vi "Run.vi"(7 "Team Index":i32, 8 "Column":i32, 9 "Row":i32, 10 "View":i32[](array[numeric]) caption="View (Team Index, -1: empty)", 11 "Runner in":refnum<class "AntFarm_MB.lvclass">) -> (0 "Replicated":refnum<class "Square.lvclass">, 1 "Direction":T1, 2 "Action":T2, 3 "Square Out":refnum<class "Square.lvclass">)   [LabVIEW 2017, in "AntFarm_MB.lvclass"]
uses:
  AntFarm_MB.lvclass
  C:/GIT/Endigit/SquareBattle/Square/Square.lvclass
  Square/Square.lvclass
  Type Defs/Action Enum.ctl
  Type Defs/Direction Enum.ctl
  AntFarm_MB.lvclass/AntFarm_MB.ctl
  TypeDefs/Cluster_Square Data.ctl
  TypeDefs/ENUM_Position ID.ctl
  Type Defs/SB Type Defs.lvlib
panel:
  out "New View Out":i32[](array[numeric])
  # "NW\nN\nNE\nE\nSE\nS\nSW\nW"
  # "NOTICE - YOU MUST NOT REMOVE THIS NOTICE. PER THE FOLLOWING LICENSE, YOU MAY REPRODUCE THIS SOFTWARE PROVIDED YOU FOLLOW THE TERMS\nOF THE LICENSE.\n\n---BEGIN BSD LICENSE (http://opensource.org/licenses/BSD-2-Clause)---\nCopyright (c) 2015, Endigit, Inc. <robert@endigit.com>\nAll rights reserved.\n\nRedistribution and use in source and binary forms, with or without modification, are permitted provided that the following conditions are met:\n\n1. Redistributions of source code must retain the above copyright notice, this list of conditions and the following disclaimer.\n\n2. Redistributions in binary form must reproduce the above copyright notice, this list of conditions and the following disclaimer in the documentation and/or other \nmaterials provided with the distribution.\n\nTHIS SOFTWARE IS PROVIDED BY THE COPYRIGHT HOLDERS AND CONTRIBUTORS \"AS IS\" AND ANY EXPRESS OR IMPLIED WARRANTIES, INCLUDING, BUT NOT \nLIMITED TO, THE IMPLIED WARRANTIES OF MERCHANTABILITY AND FITNESS FOR A PARTICULAR PURPOSE ARE DISCLAIMED. IN NO EVENT SHALL THE COPYRIGHT \nHOLDER OR CONTRIBUTORS BE LIABLE FOR ANY DIRECT, INDIRECT, INCIDENTAL, SPECIAL, EXEMPLARY, OR CONSEQUENTIAL DAMAGES (INCLUDING, BUT NOT \nLIMITED TO, PROCUREMENT OF SUBSTITUTE GOODS OR SERVICES; LOSS OF USE, DATA, OR PROFITS; OR BUSINESS INTERRUPTION) HOWEVER CAUSED AND ON \nANY THEORY OF LIABILITY, WHETHER IN CONTRACT, STRICT LIABILITY, OR TORT (INCLUDING NEGLIGENCE OR OTHERWISE) ARISING IN ANY WAY OUT OF THE USE \nOF THIS SOFTWARE, EVEN IF ADVISED OF THE POSSIBILITY OF SUCH DAMAGE.\n---END BSD LICENSE---"
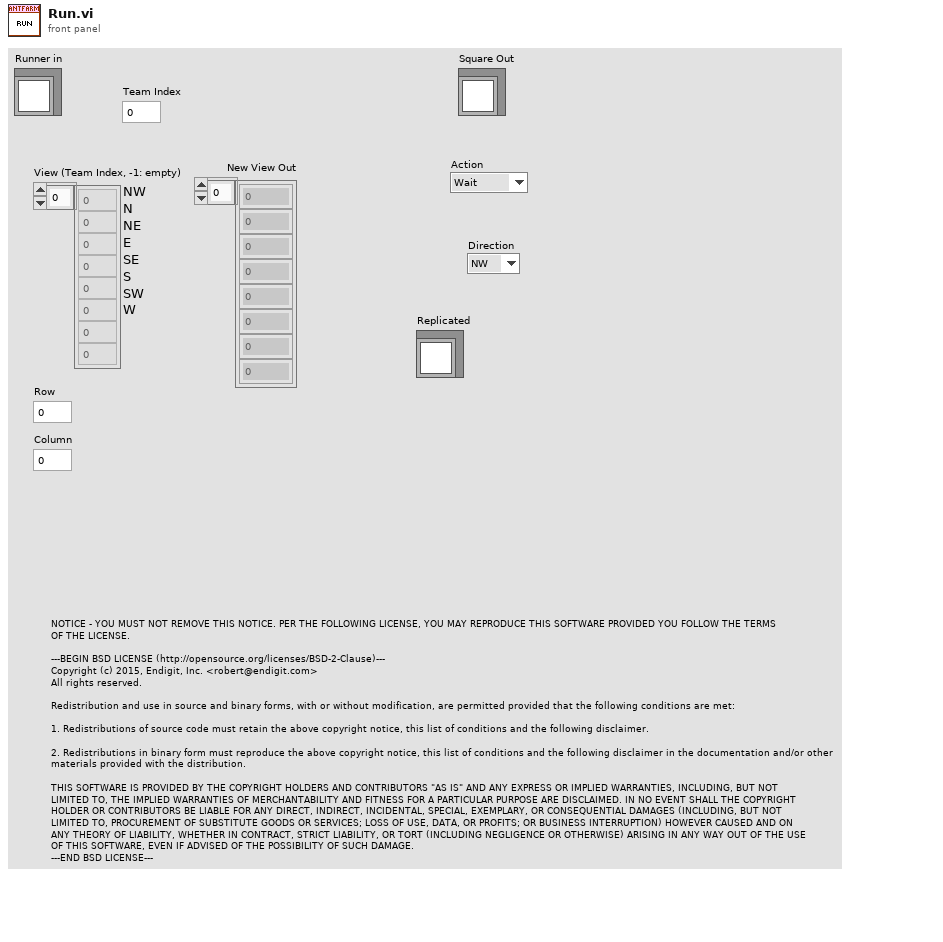
[diagram p1: front panel]
types:
  T1 = typedef "SB Type Defs.lvlib/Direction Enum.ctl" = enum16{"NW", "N", "NE", "E", "SE", "S", "SW", "W"}
  T2 = typedef "SB Type Defs.lvlib/Action Enum.ctl" = enum16{"Wait", "Move", "Attack", "Replicate"}
  T3 = typedef "Cluster_Square Data.ctl" = cluster{"Row":i32, "Column":i32, "Position ID":T4, "Primary Direction":T1, "Action":T2, "Direction":T1, "View":i32[], "New View Out":i32[], "Order ID":i32}
  T4 = typedef "ENUM_Position ID.ctl" = enum16{"0-0 Queen SW", "0-1 Path E", "0-2 Queen NW", "0-3 Path W", "1-0 Path S", "1-1 Larva SW", "1-2 Path N", "1-3 Larva NW", "2-0 Queen SE", "2-1 Path W", "2-2 Queen NE", "2-3 Path E", "3-0 Path N", "3-1 Larva SE", "3-2 Path S", "3-3 Larva NE"}
  T5 = typedef "Cluster_Ant Farm Global Data.ctl" = cluster{"Move Map":i32[][], "Danger Map":i32[][], "Attack Rows":i32[], "Attack Columns":i32[], "Square count":i32, "Last Round":i32, "Danger Threshold":i32}
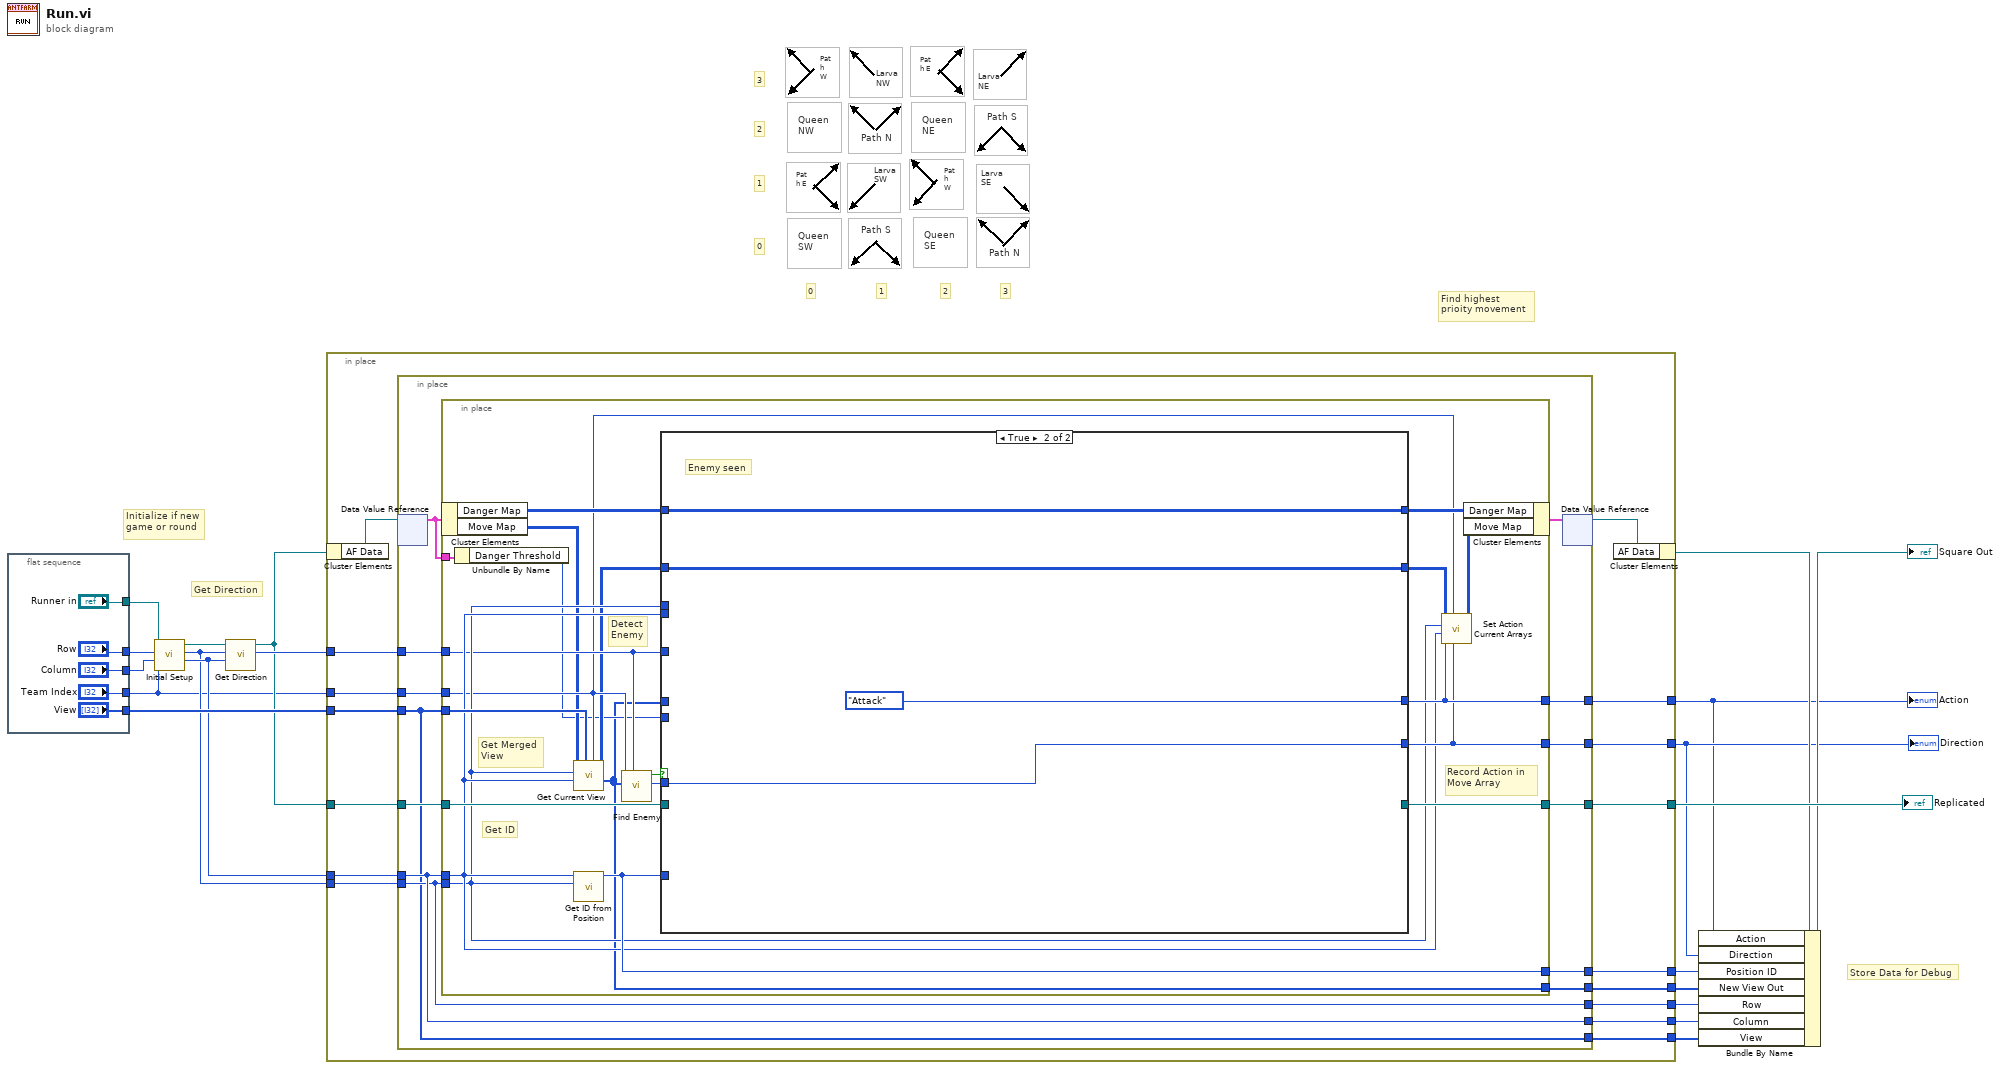
[diagram p0: block diagram]
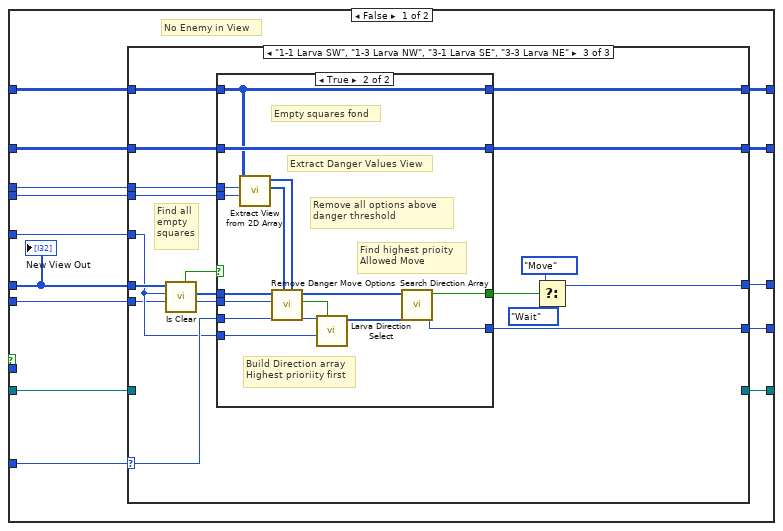
[diagram p2: hidden frame]
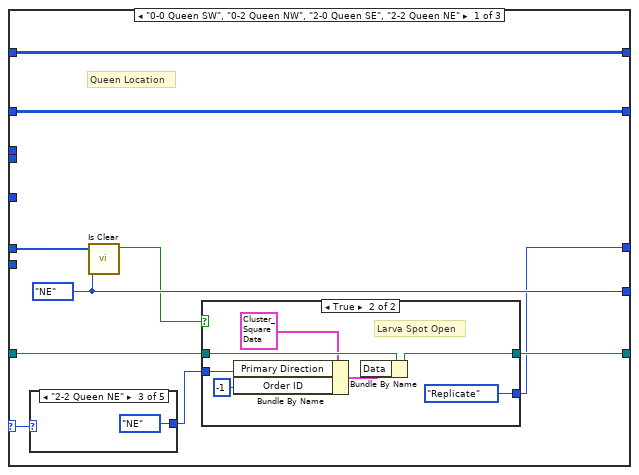
[diagram p3: hidden frame]
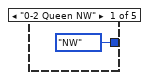
[diagram p4: hidden frame]
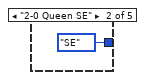
[diagram p5: hidden frame]
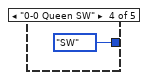
[diagram p6: hidden frame]
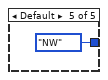
[diagram p7: hidden frame]
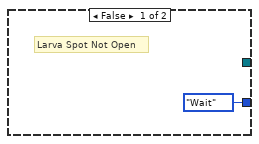
[diagram p8: hidden frame]
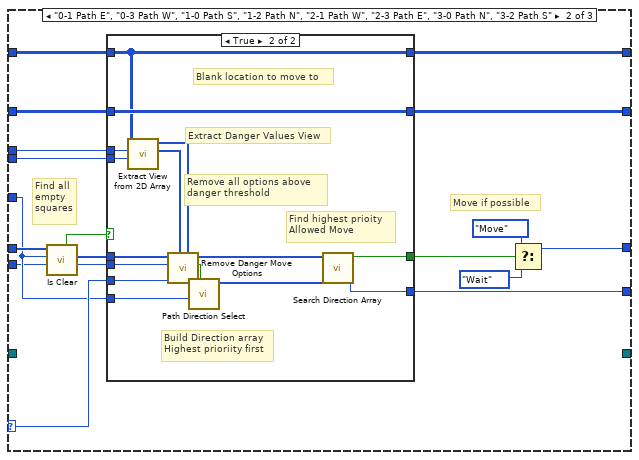
[diagram p9: hidden frame]
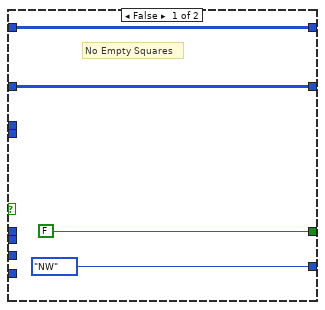
[diagram p10: hidden frame]
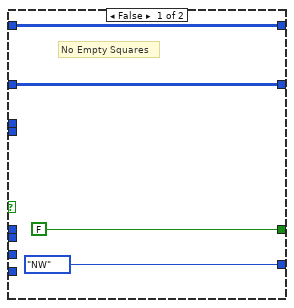
[diagram p11: hidden frame]
diagram:
  # "Store Data for Debug"
  # "Get Direction"
  # "Initialize if new\ngame or round"
  # "Path N"
  # "Path E"
  # "Path S"
  # "Path W"
  # "Path W"
  # "Path S"
  # "Path E"
  # "Path N"
  # "Larva\nNE"
  # "Larva\nSW"
  # "Larva\nNW"
  # "Queen\nNW"
  # "Queen\nNE"
  # "Queen\nSE"
  # "Larva\nSE"
  # "3"
  # "2"
  # "1"
  # "0"
  # "3"
  # "2"
  # "1"
  # "0"
  # "Find highest\nprioity movement"
  # "Queen\nSW"
  n1 = flat-sequence {
    tunnel: ["Team Index"] -> w3
    tunnel: ["View"] -> w19
    tunnel: ["Runner in"] -> w18
    tunnel: ["Row"] -> w5
    tunnel: ["Column"] -> w4
    frame #0 {
    }
  }
  n2 = call "Initial Setup.vi"("Team Index"=w3, "Column"=w4, "Row"=w5, "Runner"=w18) -> ("Column Out"=w7:i32, "Row Out"=w6:i32, "Runner Out"=w9:refnum<class "AntFarm_MB.lvclass">)  [unwired: 5 in]
  n3 = call "Get Direction.vi"("Column"=w7, "Row"=w6, "AntFarm_MB"=w9) -> ("Direction Out"=w10:T1, "AntFarm_MB Out"=w8:refnum<class "AntFarm_MB.lvclass">)  [unwired: 7 in]
  n4 = in-place {
    in-place-border: [w41] -> w20
    in-place-border: w7 -> [w40]
    in-place-border: w6 -> [w39]
    in-place-border: w3 -> [w38]
    in-place-border: w19 -> [w37]
    in-place-border: [w36] -> w11
    in-place-border: [w35] -> w12
    in-place-border: w8 -> [w34]
    in-place-border: [w33] -> w15
    in-place-border: [w32] -> w1
    in-place-border: [w31] -> w2
    in-place-border: [w30] -> w14
    in-place-border: [w29] -> w13
    in-place-border: w10 -> [w26]
    n5 = in-place-cluster #1(w8) -> ("AF Data"=w28:refnum<data-value>)
    n6 = in-place {
      in-place-border: [w54] -> w41
      in-place-border: w40 -> [w47]
      in-place-border: w39 -> [w46]
      in-place-border: w38 -> [w53]
      in-place-border: w37 -> [w43]
      in-place-border: [w52] -> w36
      in-place-border: [w51] -> w35
      in-place-border: w34 -> [w48]
      in-place-border: [w50] -> w33
      in-place-border: [w46] -> w32
      in-place-border: [w47] -> w31
      in-place-border: [w49] -> w30
      in-place-border: [w43] -> w29
      in-place-border: w26 -> [w44]
      n7 = in-place-dvr #2(w28) -> (w42:T5)  [unwired: 1 out]
      n8 = in-place {
        in-place-border: [w73] -> w54
        in-place-border: w53 -> [w60]
        in-place-border: [w72] -> w52
        in-place-border: [w71] -> w51
        in-place-border: [w69] -> w50
        in-place-border: [w55] -> w49
        in-place-border: w43 -> [w68]
        in-place-border: w48 -> [w67]
        in-place-border: w47 -> [w66]
        in-place-border: w46 -> [w65]
        in-place-border: w44 -> [w61]
        in-place-border: w42 -> [w57]
        # "Record Action in \nMove Array"
        # "Detect\nEnemy"
        # "Get Merged\nView"
        # "Get ID"
        n9 = in-place-cluster #3(w42) -> ("Danger Map"=w64:i32[][], "Move Map"=w59:i32[][])
        n10 = Unbundle By Name(w57) -> ("Danger Threshold"=w56:i32)
        n11 = call "Get Current View.vi"("Team Index"=w60, "View"=w68, "Column"=w66, "Row"=w65, "Move Array"=w59) -> ("New View Out"=w55:i32[], "Move Array"=w58:i32[][])  [unwired: 4 in, 1 out]
        n12 = call "Get ID from Position.vi"("Row"=w65, "Column"=w66) -> ("Position ID"=w69:T4)  [unwired: 9 in]
        n13 = call "Find Enemy.vi"("Primary Direction"=w61, "View"=w55, "Team Index"=w60) -> ("Direction"=w74:T1, "Found"=w75:bool)  [unwired: 7 in]
        n14 = case shown="True" w75 {
          tunnel: [w88 Action_Enum."Attack" ("Action")] -> w72
          tunnel: w74 -> [_ w188]
          tunnel: [w89 w188] -> w71
          tunnel: w55 -> [w86 _]
          tunnel: [w87 _] -> w73
          tunnel: w58 -> [w85 w186]
          tunnel: w67 -> [w84 _]
          tunnel: [w83 w186] -> w70
          tunnel: w69 -> [w82 _]
          tunnel: w61 -> [w81 _]
          tunnel: w64 -> [w80 w185]
          tunnel: [w79 w185] -> w62
          tunnel: w66 -> [w78 _]
          tunnel: w65 -> [w77 _]
          tunnel: w56 -> [w76 _]
          frame False {
            # "No Enemy in View"
            n15 = case shown="\"1-1 Larva SW\", \"1-3 Larva NW\", \"3-1 Larva SE\", \"3-3 Larva NE\"" w82 {
              selector: w82 -> [w92 w123 w159]
              tunnel: w86 -> [w99 w129 w165]
              tunnel: [w97 w121 w157] -> w89
              tunnel: [w95 w122 w158] -> w88
              tunnel: [w98 _ _] -> w87
              tunnel: w85 -> [w93 w117 w153]
              tunnel: w84 -> [w94 _ _]
              tunnel: [w93 w116 w152] -> w83
              tunnel: w81 -> [_ w120 w156]
              tunnel: w80 -> [w90 w119 w155]
              tunnel: [w90 w118 w154] -> w79
              tunnel: w78 -> [_ w115 w151]
              tunnel: w77 -> [_ w114 w150]
              tunnel: w76 -> [_ w113 w149]
              frame "0-0 Queen SW", "0-2 Queen NW", "2-0 Queen SE", "2-2 Queen NE" {
                w97 = Direction_Enum."NE" ("Primary Direction")
                # "Queen Location"
                n16 = case shown="\"2-2 Queen NE\"" w92 {
                  tunnel: [Direction_Enum."NW" ("Primary Direction") Direction_Enum."SE" ("Primary Direction") Direction_Enum."NE" ("Primary Direction") Direction_Enum."SW" ("Primary Direction") Direction_Enum."NW" ("Primary Direction")] -> w91
                  frame "0-2 Queen NW" {
                  }
                  frame "2-0 Queen SE" {
                  }
                  frame "2-2 Queen NE" {
                  }
                  frame "0-0 Queen SW" {
                  }
                  frame Default {
                  }
                }
                n17 = call "Is Clear.vi"("Primary Direction"=w97, "View"=w99) -> ("Primary Clear Out"=w96:bool)  [unwired: 7 in, 2 out]
                n18 = case shown="True" w96 {
                  tunnel: [_ w112] -> w98
                  tunnel: w91 -> [_ w107]
                  tunnel: [Action_Enum."Wait" ("Action") Action_Enum."Replicate" ("Action")] -> w95
                  tunnel: w94 -> [_ w110]
                  frame False {
                    # "Larva Spot Not Open"
                  }
                  frame True {
                    # "Larva Spot Open"
                    n19 = Bundle By Name(cluster=T3 {"Row"=0, "Column"=0, "Position ID"=enum."0-0 Queen SW", "Primary Direction"=enum."NW", "Action"=enum."Wait", "Direction"=enum."NW", "View"=[], "New View Out"=[], "Order ID"=0} ("Data"), "Primary Direction"=w107, "Order ID"=-1) -> (w108:T3)
                    n20 = Bundle By Name(cluster=w110, "Data"=w108) -> (w112:refnum<class "AntFarm_MB.lvclass">)
                  }
                }
              }
              frame "0-1 Path E", "0-3 Path W", "1-0 Path S", "1-2 Path N", "2-1 Path W", "2-3 Path E", "3-0 Path N", "3-2 Path S" {
                # "Find all\nempty\nsquares"
                # "Move if possible"
                n21 = call "Is Clear.vi"("Primary Direction"=w120, "View"=w129) -> ("Clear Array Out"=w127:T1[], "Found Out"=w128:bool)  [unwired: 7 in, 1 out]
                n22 = case shown="True" w128 {
                  tunnel: w127 -> [_ w138]
                  tunnel: [Direction_Enum."NW" ("Seconday Move Direction Out") w147] -> w121
                  tunnel: [FALSE w146] -> w126
                  tunnel: w123 -> [_ w148]
                  tunnel: w120 -> [_ w145]
                  tunnel: [w131 w143] -> w118
                  tunnel: w119 -> [w131 w143]
                  tunnel: w117 -> [w130 w144]
                  tunnel: [w130 w144] -> w116
                  tunnel: w115 -> [_ w134]
                  tunnel: w114 -> [_ w142]
                  tunnel: w113 -> [_ w139]
                  frame False {
                    # "No Empty Squares"
                  }
                  frame True {
                    # "Blank location to move to"
                    # "Build Direction array\nHighest prioriity first"
                    # "Extract Danger Values View"
                    # "Find highest prioity \nAllowed Move"
                    # "Remove all options above \ndanger threshold"
                    n23 = call "Extract View from 2D Array.vi"("Column"=w134, "Row"=w142, "Board Array"=w143) -> ("View Out"=w141:i32[], "Directions Out"=w140:T1[])  [unwired: 7 in]
                    n24 = call "Remove Danger Move Options.vi"("Danger Directions"=w140, "Danger View"=w141, "Danger Threshold"=w139, "Direction List"=w138) -> ("Danger"=w135:bool, "Safe Directions Out"=w137:T1[])  [unwired: 6 in]
                    n25 = call "Path Direction Select.vi"("Danger"=w135, "Target Direction"=w145, "Position ID"=w148) -> ("Direction Array"=w136:T1[])  [unwired: 8 in]
                    n26 = call "Search Direction Array.vi"("Target Items"=w136, "Search Array"=w137) -> ("Found Direction"=w147:T1, "Found"=w146:bool)  [unwired: 8 in]
                  }
                }
                n27 = Select(t=Action_Enum."Move" ("Action"), s=w126, f=Action_Enum."Wait") -> (s? t:f=w122:T2)
              }
              frame "1-1 Larva SW", "1-3 Larva NW", "3-1 Larva SE", "3-3 Larva NE" {
                # "Find all\nempty\nsquares"
                n28 = call "Is Clear.vi"("Primary Direction"=w156, "View"=w165) -> ("Clear Array Out"=w163:T1[], "Found Out"=w164:bool)  [unwired: 7 in, 1 out]
                n29 = case shown="True" w164 {
                  tunnel: w163 -> [_ w175]
                  tunnel: [Direction_Enum."NW" ("Seconday Move Direction Out") w182] -> w157
                  tunnel: [FALSE w181] -> w162
                  tunnel: w159 -> [_ w184]
                  tunnel: w156 -> [_ w183]
                  tunnel: w155 -> [w166 w179]
                  tunnel: [w166 w179] -> w154
                  tunnel: [w167 w180] -> w152
                  tunnel: w153 -> [w167 w180]
                  tunnel: w151 -> [_ w171]
                  tunnel: w150 -> [_ w178]
                  tunnel: w149 -> [_ w170]
                  frame False {
                    # "No Empty Squares"
                  }
                  frame True {
                    # "Find highest prioity \nAllowed Move"
                    # "Build Direction array\nHighest prioriity first"
                    # "Remove all options above \ndanger threshold"
                    # "Extract Danger Values View"
                    # "Empty squares fond"
                    n30 = call "Extract View from 2D Array.vi"("Column"=w171, "Row"=w178, "Board Array"=w179) -> ("View Out"=w177:i32[], "Directions Out"=w176:T1[])  [unwired: 7 in]
                    n31 = call "Remove Danger Move Options.vi"("Danger Directions"=w176, "Danger View"=w177, "Danger Threshold"=w170, "Direction List"=w175) -> ("Danger"=w172:bool, "Safe Directions Out"=w174:T1[])  [unwired: 6 in]
                    n32 = call "Larva Direction Select.vi"("Danger"=w172, "Target Direction"=w183, "Position ID"=w184) -> ("Move Array Out"=w173:T1[])  [unwired: 8 in]
                    n33 = call "Search Direction Array.vi"("Target Items"=w173, "Search Array"=w174) -> ("Found Direction"=w182:T1, "Found"=w181:bool)  [unwired: 8 in]
                  }
                }
                n34 = Select(t=Action_Enum."Move" ("Action"), s=w162, f=Action_Enum."Wait") -> (s? t:f=w158:T2)
              }
            }
            "New View Out" <- w86
          }
          frame True {
            # "Enemy seen"
          }
        }
        n35 = call "Set Action Current Arrays.vi"("Direction"=w71, "Team Index"=w60, "Action"=w72, "Column"=w66, "Row"=w65, "MoveTrack"=w70) -> ("MoveTrack Out"=w63:i32[][])  [unwired: 5 in]
        n36 = in-place-cluster #3("Danger Map"=w62, "Move Map"=w63) -> (w45:T5)
      }
      n37 = in-place-dvr #2(w45) -> (w27:refnum<data-value>)  [unwired: 1 out]
    }
    n38 = in-place-cluster #1("AF Data"=w27) -> (w17:refnum<class "AntFarm_MB.lvclass">)
  }
  "Action" <- w11
  "Direction" <- w12
  "Replicated" <- w20
  n39 = Bundle By Name(cluster=w17, "Action"=w11, "Direction"=w12, "Position ID"=w15, "New View Out"=w14, "Row"=w1, "Column"=w2, "View"=w13) -> (→"Square Out":refnum<class "AntFarm_MB.lvclass">)
